vi "PLCtoGUIint.vi"(9 "DB Val Qty":u16, 11 "DB Input Vals":u8[](array[numeric])=[0, 0, 0, 0]) -> (3 "RealValue":i16[](array[numeric]))   [LabVIEW 2023]
panel:
  out "Array":bool[](array[boolean])
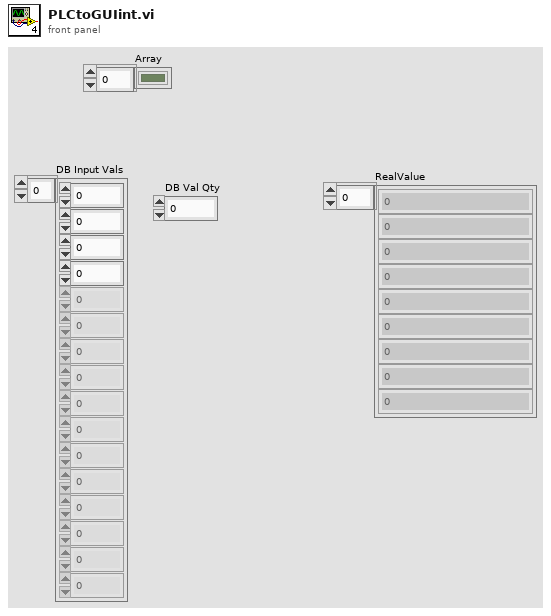
[diagram p1: front panel]
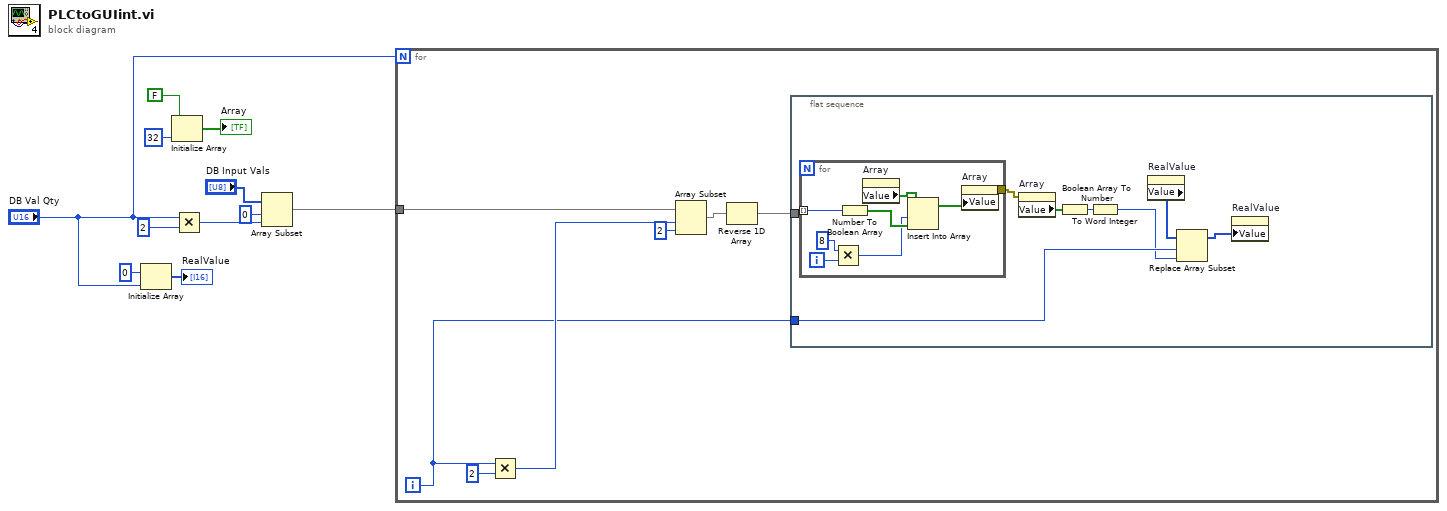
[diagram p0: block diagram]
diagram:
  n1 = Initialize Array(i16 0 ("element"), "DB Val Qty") -> (→"RealValue":i16[])
  n2 = Initialize Array(FALSE, 32 ("dimension size")) -> (→"Array":bool[])
  n3 = Multiply(x="DB Val Qty", y=u8 2) -> (x*y=w6:u16)
  n4 = Array Subset(array="DB Input Vals", index=0, length=w6) -> (w8:u8[])
  n5 = for {
    N: "DB Val Qty" -> [_]
    tunnel: w8 -> [w17]
    i -> [w12]
    n6 = Multiply(x=w12, y=2) -> (x*y=w16:i32)
    n7 = Array Subset(array=w17, index=w16, length=2) -> (w13:u8[])
    n8 = Reverse 1D Array(array=w13) -> (reversed array=w14:u8[])
    n9 = flat-sequence {
      tunnel: w14 -> [w26]
      tunnel: w12 -> [w22]
      frame #0 {
        n10 = for {
          tunnel: w26 -> [w32] mode=indexing
          tunnel: [w27] -> w21
          i -> [w30]
          n11 = Multiply(x=8, y=w30) -> (x*y=w28:i32)
          n12 = Number To Boolean Array(number=w32) -> (Boolean array=w33:bool[])
          n13 = property on="Array" class="Arr (strict)"() -> ("Value"=w34:bool[])  [unwired: 2 in, 2 out]
          n14 = Insert Into Array(array=w34, index=w28, new element=w33) -> (w31:bool[])
          n15 = property on="Array" class="Arr (strict)"("Value"=w31) -> (error out=w27:errorcluster)  [unwired: 2 in, 1 out]
        }
        n16 = property on="Array" class="Arr (strict)"(error in=w21) -> ("Value"=w23:bool[])  [unwired: 1 in, 2 out]
        n17 = Boolean Array To Number(Boolean array=w23) -> (number=w20:u32)
        n18 = To Word Integer(number=w20) -> (16bit integer=w19:i16)
        n19 = property on="RealValue" class="Arr (strict)"() -> ("Value"=w24:i16[])  [unwired: 2 in, 2 out]
        n20 = Replace Array Subset(array=w24, new element=w19, index=w22) -> (w25:i16[])
        n21 = property on="RealValue" class="Arr (strict)"("Value"=w25) -> ()  [unwired: 2 in, 2 out]
      }
    }
  }
